vi "lsl destroy inlet.vi"(8 "error in (no error)":errorcluster, 11 "in":cluster{}) -> (0 "error out":errorcluster, 3 "in out":cluster{})   [LabVIEW 2018, in "liblsl-LabVIEW.lvlib"]
doc: "extern LIBLSL_C_API void lsl_destroy_inlet(lsl_inlet in);"
uses:
  <userlib>/liblsl-LabVIEW/liblsl-LabVIEW.lvlib
  <userlib>/liblsl-LabVIEW/liblsl64.dll
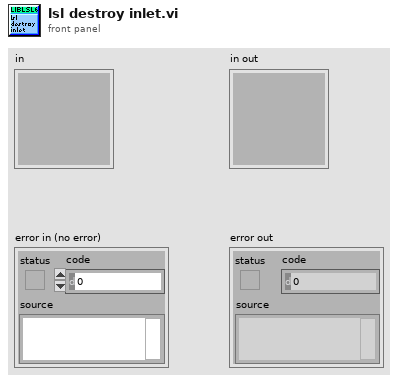
[diagram p1: front panel]
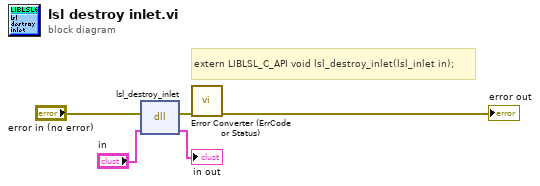
[diagram p0: block diagram]
diagram:
  # "extern LIBLSL_C_API void lsl_destroy_inlet(lsl_inlet in);"
  n1 = dll-call lib="C:/Program Files/National Instruments/LabVIEW 2018/user.lib/liblsl-LabVIEW/liblsl64.*" fn="lsl_destroy_inlet"(error in="error in (no error)", "in"="in") -> (error out=w2:errorcluster, "in"=→"in out":cluster{})  [unwired: 3 in, 1 out]
  n2 = call <userlib>:"Error Converter (ErrCode or Status).vi"("error in (no error)"=w2) -> ("error out"=→"error out":errorcluster)  [unwired: 10 in]
